vi "initialize.vi"(11 "path in":path=path "hl2ss_ulm.dll") -> (2 "error":bool, 3 "path out":path)   [LabVIEW 2023]
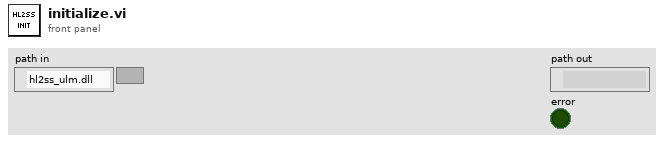
[diagram p1: front panel]
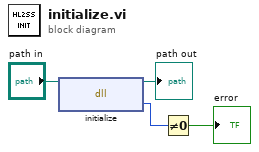
[diagram p0: block diagram]
diagram:
  n1 = dll-call lib="C:/Users/jcds/Documents/GitHub/hl2ss/extensions/client_labview/hl2ss_ulm.dll" fn="initialize"(path in="path in") -> (path out=→"path out":path, "return type"=w2:i32)  [unwired: 2 in, 1 out]
  n2 = Not Equal To 0?(x=w2) -> (x != 0?=→"error":bool)
